vi "Stepper Command.vi"(0 "Instrument Address":refnum<visa-resource-name>, 1 "Motor Number":u32=1 min=1 max=255 step=1, 2 "Command":string, 3 "Mode":bool, 4 "Timeout Limit":sgl=0.1 format="%.2f", 5 "error in (no error)":errorcluster) -> (6 "Timeout":bool, 7 "Response":string, 8 "error out":errorcluster)   [LabVIEW 2021]
uses:
  Serial Support VISA.llb/Serial Actions.ctl
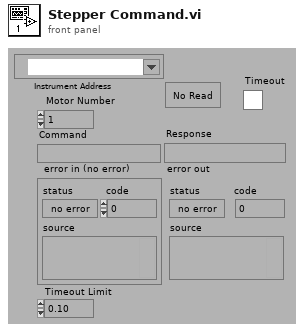
[diagram p1: front panel]
types:
  T1 = typedef "Serial Actions.ctl" = enum16{"Init", "Break", "Clear Buffer", "Write", "Read", "N Bytes", "Lock", "Unlock", "Close"}
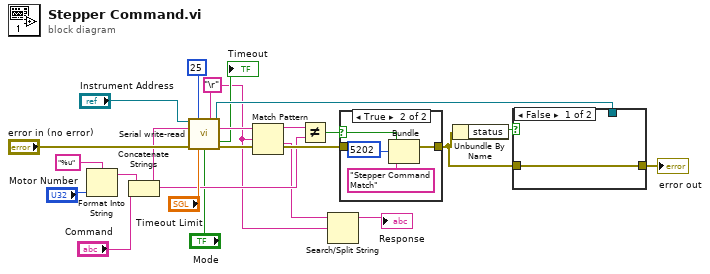
[diagram p0: block diagram]
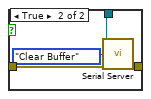
[diagram p2: hidden frame]
diagram:
  w3 = "\r" ("EOT Chars (cr/lf)")
  n1 = Format Into String(format string="%u", "Motor Number") -> (resulting string=w17:string)  [unwired: 2 in, 1 out]
  n2 = Concatenate Strings(w17, "Command") -> (w12:string)
  n3 = call "Serial write-read.vi"("VISA Resource Name"="Instrument Address", "Max Char to Read"=u32 25, "EOT Chars (cr/lf)"=w3, "String To Send"=w12, "error in (no error)"="error in (no error)", "Timeout Limit"="Timeout Limit", "Read Echo?"="Mode") -> ("dup VISA Resource Name"=w10:refnum<visa-resource-name>, "Serial Read"=w8:string, "Timeout"=→"Timeout":bool, "error out"=w15:errorcluster)  [unwired: 3 in, 2 out]
  n4 = Match Pattern(string=w8, regular expression=w3) -> (before substring=w7:string, after substring=w5:string)  [unwired: 1 in, 2 out]
  n5 = Not Equal?(x=w7, y=w12) -> (x != y?=w22:bool)
  n6 = Search/Split String(string=w5, search string/char (-)=w3) -> (substring before match=→"Response":string)  [unwired: 1 in, 2 out]
  n7 = case shown="True" w22 {
    selector: w22 -> [_ w26]
    tunnel: [w23 w27] -> w1
    tunnel: w15 -> [w23 _]
    frame False {
    }
    frame True {
      n8 = Bundle(w26, 5202, "Stepper Command Match") -> (w27:errorcluster)  [unwired: 1 in]
    }
  }
  n9 = Unbundle By Name(w1) -> ("status"=w16:bool)
  n10 = case shown="False" w16 {
    tunnel: w10 -> [_ w31]
    tunnel: [w28 w30] -> w2
    tunnel: w1 -> [w28 w29]
    frame False {
    }
    frame True {
      n11 = call "Serial Server.vi"("VISA Resource Name"=w31, "Action"=Serial_Actions."Clear Buffer", "error in (no error)"=w29) -> ("error out"=w30:errorcluster)  [unwired: 8 in, 4 out]
    }
  }
  "error out" <- w2
